vi "Pop Up.vi"(11 "Ex Queue Actor in":refnum<class "Ex Queue Actor.lvclass">) -> (3 "Ex Queue Actor out":refnum<class "Ex Queue Actor.lvclass">)   [LabVIEW 2021, in "Ex Queue Actor.lvlib" / "Ex Queue Actor.lvclass"]
uses:
  Ex Queue Actor.lvclass
  Actor/Queue Actor/Queue Actor.lvclass
  Actor/Msgs/Queue Create/Queue Create Msg/Queue Create Msg.lvclass
  C:/git/jettl/src/Actor/Msg/Msg.lvclass
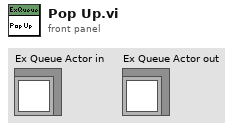
[diagram p1: front panel]
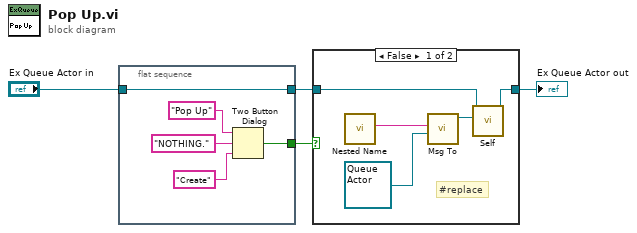
[diagram p0: block diagram]
diagram:
  n1 = flat-sequence {
    tunnel: [w9] -> w1
    tunnel: "Ex Queue Actor in" -> [w9]
    tunnel: [w6] -> w3
    frame #0 {
      n2 = Two Button Dialog(message="Pop Up", 1:"Create" ("F button name (\"Cancel\")"), 2:"NOTHING." ("T button name (\"OK\")")) -> (T button?=w6:bool)
    }
  }
  n3 = case shown="False" w3 {
    tunnel: w1 -> [w14 w15]
    tunnel: [w13 w15] -> w2
    frame False {
      # "#replace"
      n4 = call "Nested Name.vi"() -> ("Nested Name"=w11:string)  [unwired: 11 in]
      n5 = call "Msg To.vi"("Queue Actor"=refnum<class "Queue Actor.lvclass"> refnum, "Alias"=w11) -> ("Queue Create Msg out"=w12:refnum<class "Queue Create Msg.lvclass">)  [unwired: 9 in]
      n6 = call-dynamic "Self.vi"("Msg"=w12, "Ex Queue Actor in"=w14) -> ("Ex Queue Actor out"=w13:refnum<class "Ex Queue Actor.lvclass">)  [unwired: 9 in]
    }
    frame True {
    }
  }
  "Ex Queue Actor out" <- w2
